vi "VCS Get Homing Parameter.vi"(8 "error in (no error)":errorcluster, 11 "axis in":cluster{"keyHandle":u32, "nodeId":u16}={"keyHandle"=0, "nodeId"=1}) -> (0 "error out":errorcluster, 2 "homingParameter":T1, 3 "axis out":cluster{"keyHandle":u32, "nodeId":u16}={"keyHandle"=0, "nodeId"=1})   [LabVIEW 2010]
doc: "<B>VCS Get Homing Parameter</B> reads all homing parameters."
uses:
  Resources/EposCmd.dll
  Resources/EposCmd64.dll
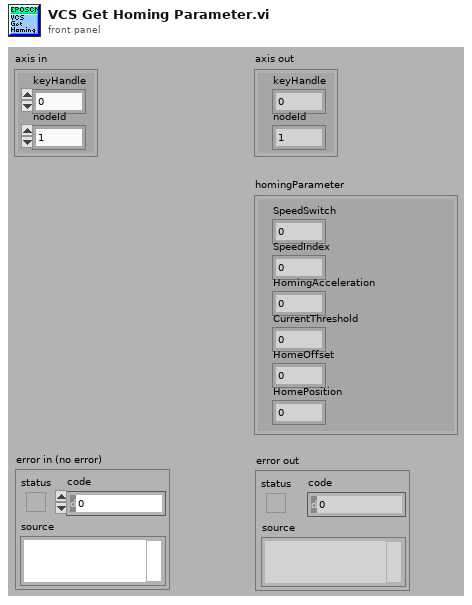
[diagram p1: front panel]
types:
  T1 = cluster{"SpeedSwitch":u32, "SpeedIndex":u32, "HomingAcceleration":u32, "CurrentThreshold":u16, "HomeOffset":i32, "HomePosition":i32}
  T2 = cluster{"pSpeedSwitch":u32, "pSpeedIndex":u32, "pHomingAcceleration":u32, "pCurrentThreshold":u16, "pHomeOffset":i32, "pHomePosition":i32}
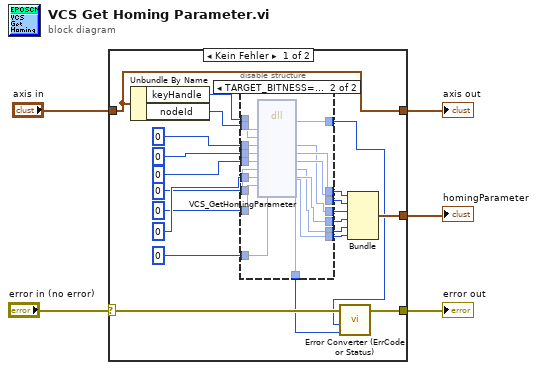
[diagram p0: block diagram]
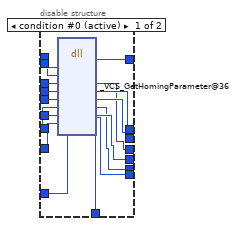
[diagram p2: hidden frame]
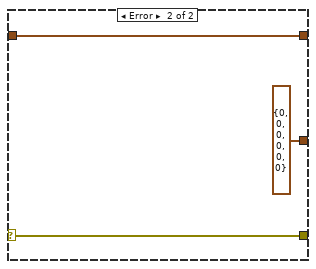
[diagram p3: hidden frame]
diagram:
  n1 = case shown="Kein Fehler" "error in (no error)" {
    selector: "error in (no error)" -> [w26 w63]
    tunnel: [w25 w63] -> w4
    tunnel: "axis in" -> [w21 w62]
    tunnel: [w21 w62] -> w2
    tunnel: [w7 T2 {"pSpeedSwitch"=0, "pSpeedIndex"=0, "pHomingAcceleration"=0, "pCurrentThreshold"=0, "pHomeOffset"=0, "pHomePosition"=0}] -> w1
    frame No Error {
      n2 = Unbundle By Name(w21) -> ("keyHandle"=w23:u32, "nodeId"=w22:u16)
      n3 = disable-structure shown="TARGET_BITNESS==64" {
        disable-tunnel: [w43 w60] -> w24
        disable-tunnel: w23 -> [w42 w59]
        disable-tunnel: w22 -> [w41 w58]
        disable-tunnel: u32 0 ("pHomingAcceleration") -> [w40 w57]
        disable-tunnel: u32 0 ("pSpeedSwitch") -> [w39 w56]
        disable-tunnel: u32 0 ("pSpeedIndex") -> [w38 w55]
        disable-tunnel: u16 0 ("pCurrentThreshold") -> [w37 w54]
        disable-tunnel: 0 ("pHomeOffset") -> [w36 w53]
        disable-tunnel: 0 ("pHomePosition") -> [w35 w52]
        disable-tunnel: u32 0 ("pErrorCode") -> [w34 w51]
        disable-tunnel: [w33 w50] -> w13
        disable-tunnel: [w32 w49] -> w12
        disable-tunnel: [w31 w48] -> w11
        disable-tunnel: [w30 w47] -> w10
        disable-tunnel: [w29 w46] -> w9
        disable-tunnel: [w28 w45] -> w8
        disable-tunnel: [w27 w44] -> w6
        frame condition #0 (active) {
          n4 = dll-call lib="C:/Sources/LabView/maxon EPOS/Resources/EposCmd.*" fn="_VCS_GetHomingParameter@36"("KeyHandle"=w42, "NodeId"=w41, "pHomingAcceleration"=w40, "pSpeedSwitch"=w39, "pSpeedIndex"=w38, "pHomeOffset"=w36, "pCurrentThreshold"=w37, "pHomePosition"=w35, "pErrorCode"=w34) -> (w27:i32, "pHomingAcceleration"=w31:u32, "pSpeedSwitch"=w33:u32, "pSpeedIndex"=w32:u32, "pHomeOffset"=w29:i32, "pCurrentThreshold"=w30:u16, "pHomePosition"=w28:i32, "pErrorCode"=w43:u32)  [unwired: 5 in, 2 out]
        }
        frame condition #1 {
          n5 = dll-call lib="C:/setup/Resources/EposCmd64.*" fn="VCS_GetHomingParameter" ("EposCmd.dll:_VCS_GetHomingParameter@36")("KeyHandle"=w59, "NodeId"=w58, "pHomingAcceleration"=w57, "pSpeedSwitch"=w56, "pSpeedIndex"=w55, "pHomeOffset"=w53, "pCurrentThreshold"=w54, "pHomePosition"=w52, "pErrorCode"=w51) -> ("Rückgabetyp"=w44:i32, "pHomingAcceleration"=w48:u32, "pSpeedSwitch"=w50:u32, "pSpeedIndex"=w49:u32, "pHomeOffset"=w46:i32, "pCurrentThreshold"=w47:u16, "pHomePosition"=w45:i32, "pErrorCode"=w60:u32)  [unwired: 5 in, 2 out]
        }
      }
      n6 = call "Error Converter (ErrCode or Status).vi"("error code"=w24, "return type"=w6, "error in (no error)"=w26) -> ("error out"=w25:errorcluster)  [unwired: 7 in]
      n7 = Bundle("pSpeedSwitch"=w13, "pSpeedIndex"=w12, "pHomingAcceleration"=w11, "pCurrentThreshold"=w10, "pHomeOffset"=w9, "pHomePosition"=w8) -> (w7:T2)  [unwired: 1 in]
    }
    frame Error {
    }
  }
  "error out" <- w4
  "homingParameter" <- w1
  "axis out" <- w2
